vi "FL_Reshape_data_for_memory_storage_(strings).vi"(1 "DEC string input":string[][](array[string])) -> (0 "DEC string output":string[](array[string]))   [LabVIEW 2018, in "Tracker.lvlib"]
uses:
  Tracker.lvlib
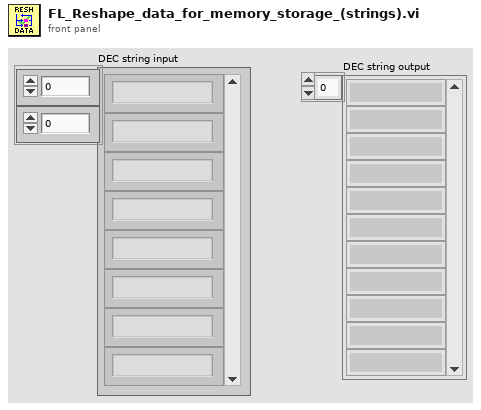
[diagram p1: front panel]
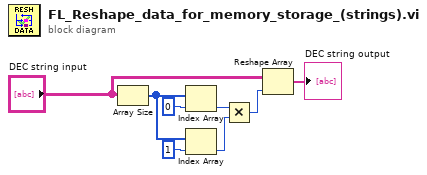
[diagram p0: block diagram]
diagram:
  n1 = Array Size(array="DEC string input") -> (size(s)=w6:i32[])
  n2 = Index Array(array=w6, index=0) -> (element=w5:i32)
  n3 = Index Array(array=w6, index=1) -> (element=w4:i32)
  n4 = Multiply(x=w5, y=w4) -> (x*y=w3:i32)
  n5 = Reshape Array("DEC string input", w3) -> (→"DEC string output":string[])
